vi "Menu Item Selected.vi"(8 "error in (no error)":errorcluster, 9 "Menu Item":string, 11 "module in":refnum<class "Header.lvclass">) -> (0 "error out":errorcluster, 3 "module out":refnum<class "Header.lvclass">)   [LabVIEW 2024, in "Header.lvclass"]
uses:
  Header.lvclass
  Header.lvclass/Header.ctl
  JQMHCore/Module/RQMHModule.lvclass
  Menu Item Selected.ctl
  C:/Github/JQMH/JQMHCore/Module/RQMHModule.lvclass
  C:/Github/JQMH/ModuleTemplates/Header/Header.lvclass
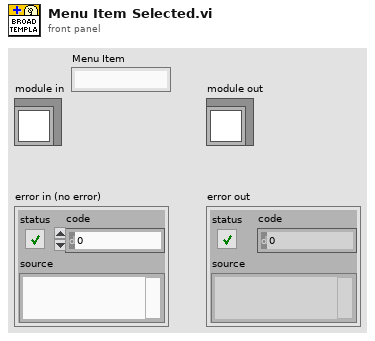
[diagram p1: front panel]
types:
  T1 = typedef "Header.lvclass/Menu Item Selected.ctl" = cluster{"Module":refnum<class "RQMHModule.lvclass">, "Menu Item":string}
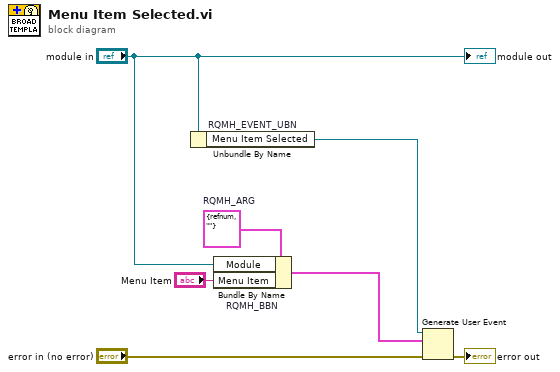
[diagram p0: block diagram]
diagram:
  w4 = T1 {"Module"=refnum, "Menu Item"=""}  # RQMH_ARG
  n1 = Unbundle By Name "RQMH_EVENT_UBN"("module in") -> ("Menu Item Selected"=w7:refnum<user-event>)
  n2 = Bundle By Name "RQMH_BBN"(cluster=w4, "Module"="module in", "Menu Item"="Menu Item") -> (w3:T1)
  n3 = Generate User Event(user event=w7, event data cluster=w3, error in="error in (no error)") -> (error out=→"error out":errorcluster)  [unwired: 1 in, 1 out]
  "module out" <- "module in"
